vi "oa_Detect Parameters Change for Overall Level.vi"(7 "reset (F)":bool, 10 "integration revolution":dbl=1.0, 11 "even angle position info":T1) -> (2 "dup integration revolution":dbl=1.0, 3 "dup even angle position":T1, 5 "reset out":bool)   [LabVIEW 2017, in "SoundVib_Resampling.lvlib"]
uses:
  <vilib>/addons/Sound and Vibration/Order Analysis/Resample Order Tracking/SoundVib_Resampling.lvlib
  <vilib>/addons/Sound and Vibration/Order Analysis/Misc/OAT Position Info.ctl
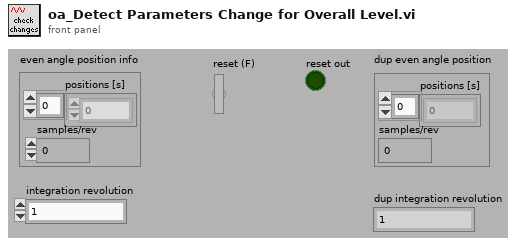
[diagram p1: front panel]
types:
  T1 = typedef "OAT Position Info.ctl" = cluster{"positions [s]":dbl[], "samples/rev":dbl}
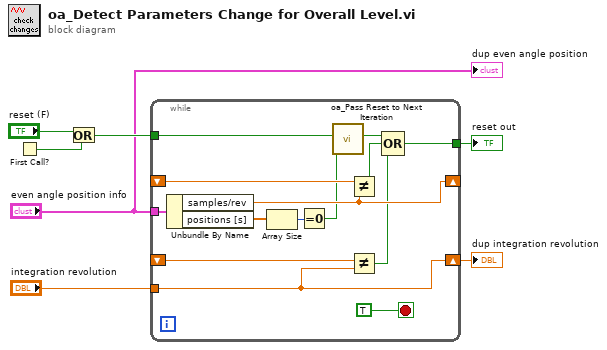
[diagram p0: block diagram]
diagram:
  n1 = First Call?() -> (First Call?: T/F=w5:bool)
  n2 = Or(x="reset (F)", y=w5) -> (x .or. y?=w4:bool)
  n3 = while {
    tunnel: "even angle position info" -> [w20]
    tunnel: "integration revolution" -> [w16]
    shift-right: [w18] -> _
    shift-left: _ -> [w19]
    shift-right: [w16] -> w2
    shift-left: _ -> [w17]
    tunnel: w4 -> [w9]
    tunnel: [w13] -> w3
    stop <- TRUE stop-if-true
    n4 = Unbundle By Name(w20) -> ("samples/rev"=w18:dbl, "positions [s]"=w12:dbl[])
    n5 = Array Size(array=w12) -> (size(s)=w11:i32)
    n6 = Equal To 0?(x=w11) -> (x = 0?=w10:bool)
    n7 = call <vilib>:"oa_Pass Reset to Next Iteration.vi"("trigger"=w10, "reset?(F)"=w9) -> ("reset out"=w8:bool)  [unwired: 9 in]
    n8 = Not Equal?(x=w19, y=w18) -> (x != y?=w15:bool)
    n9 = Not Equal?(x=w17, y=w16) -> (x != y?=w14:bool)
    n10 = Compound Arithmetic op=OR(w8, w15, w14) -> (w13:bool)
  }
  "reset out" <- w3
  "dup integration revolution" <- w2
  "dup even angle position" <- "even angle position info"
